vi "4.5.vi"() -> ()   [LabVIEW 2017]
panel:
  out "循环次数":i32
  in  "指定值":dbl
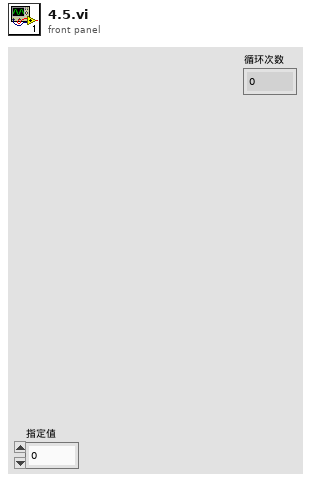
[diagram p1: front panel]
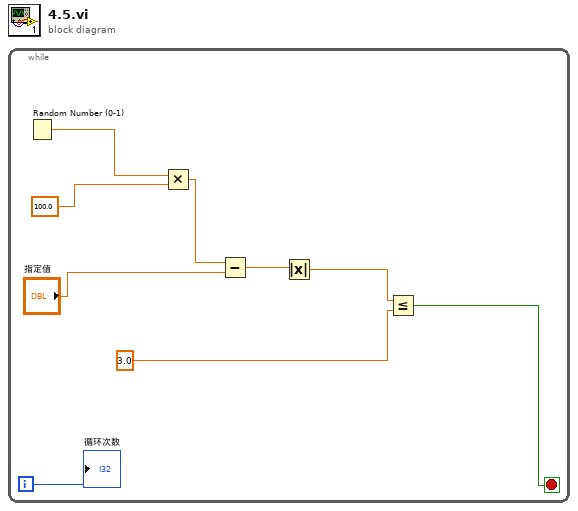
[diagram p0: block diagram]
diagram:
  n1 = while {
    i -> [w7]
    stop <- w3 stop-if-true
    n2 = Random Number (0-1)() -> (number: 0 to 1=w9:dbl)
    n3 = Multiply(x=w9, y=100.0) -> (x*y=w5:dbl)
    n4 = Subtract(x=w5, y="指定值") -> (x-y=w4:dbl)
    n5 = Absolute Value(x=w4) -> (abs(x)=w2:dbl)
    n6 = Less Or Equal?(x=w2, y=3.0) -> (x <= y?=w3:bool)
    "循环次数" <- w7
  }
